vi "Refresh To Find New VIs.vi"(8 "error in":errorcluster, 10 "VIs  to exclude":variant, 11 "state in":T1) -> (0 "error out":errorcluster, 3 "state out":T1)   [LabVIEW 2010, in "NI_SE_Config Front Panel Layout.lvlib"]
uses:
  NI_SE_Config Front Panel Layout.lvlib
  State.ctl
  VI Info.ctl
  VI Panel Layout/VI Panel Layout.lvclass
  NI_SE_Front Panel Layout.lvlib
panel:
  in  "dummy object":dbl
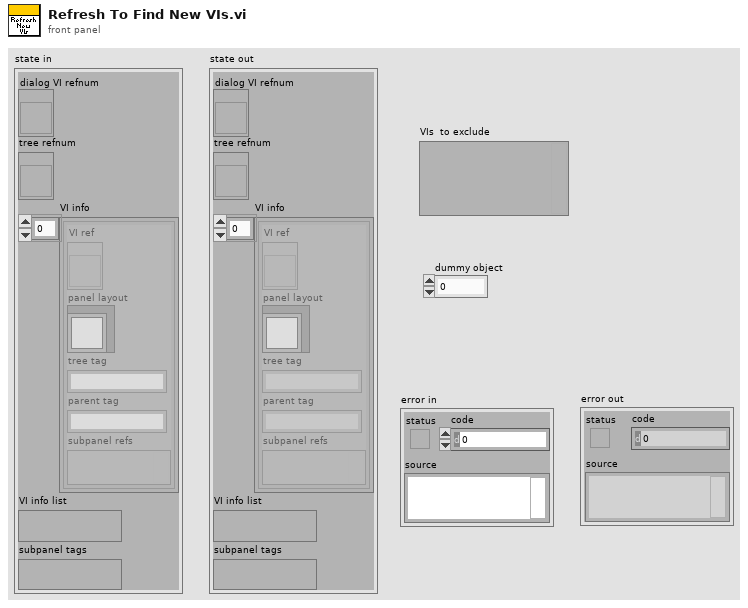
[diagram p1: front panel]
types:
  T1 = typedef "NI_SE_Config Front Panel Layout.lvlib/State.ctl" = cluster{"dialog VI refnum":refnum<vi>, "tree refnum":refnum<vi>, "VI info":T2[], "VI info list":variant, "subpanel tags":variant}
  T2 = typedef "NI_SE_Config Front Panel Layout.lvlib/VI Info.ctl" = cluster{"VI ref":refnum<vi>, "panel layout":refnum<class "VI Panel Layout.lvclass">, "tree tag":string, "parent tag":string, "subpanel refs":variant}
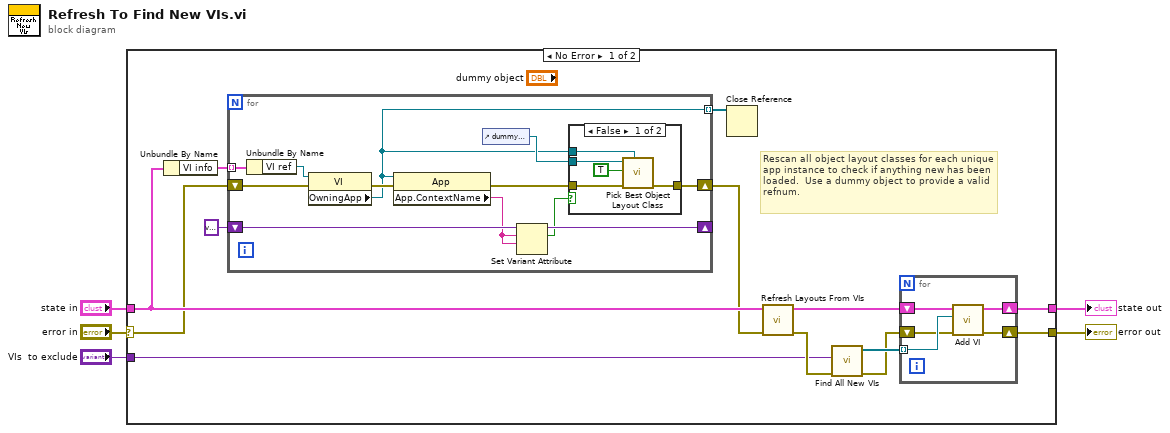
[diagram p0: block diagram]
diagram:
  n1 = case shown="No Error" "error in" {
    selector: "error in" -> [w8 w42]
    tunnel: "state in" -> [w11 w43]
    tunnel: [w13 w43] -> w3
    tunnel: [w12 w42] -> w2
    tunnel: "VIs  to exclude" -> [w14 _]
    frame No Error {
      # "Rescan all object layout classes for each unique app instance to check if anything new has been loaded.  Use a dummy object to provide a valid refnum."
      n2 = Unbundle By Name(w11) -> ("VI info"=w10:T2[])
      n3 = for {
        tunnel: w10 -> [w30] mode=indexing
        shift-right: [w28] -> _
        shift-left: variant -> [w27]
        shift-right: [w23] -> w7
        shift-left: w8 -> [w26]
        tunnel: [w19] -> w6 mode=indexing
        n4 = Unbundle By Name(w30) -> ("VI ref"=w29:refnum<vi>)
        n5 = property class="VI"(reference=w29, error in=w26) -> (error out=w22:errorcluster, "OwningApp"=w19:refnum<vi>)  [unwired: 1 out]
        n6 = property class="App"(reference=w19, error in=w22) -> (error out=w21:errorcluster, "App.ContextName"=w20:string)  [unwired: 1 out]
        n7 = control-ref of="dummy object"() -> (w24:refnum<vi>)
        n8 = Set Variant Attribute(Variant=w27, name=w20, value=w20) -> (Variant out=w28:variant, replaced=w25:bool)  [unwired: 1 in, 1 out]
        n9 = case shown="False" w25 {
          tunnel: w24 -> [w34 _]
          tunnel: w19 -> [w33 _]
          tunnel: w21 -> [w32 w36]
          tunnel: [w31 w36] -> w23
          frame False {
            n10 = call "Pick Best Object Layout Class.vi"("application reference"=w33, "error in"=w32, "rescan classes (F)"=TRUE ("rescan (F)"), "GObj Refnum"=w34) -> ("error out"=w31:errorcluster)  [unwired: 5 in, 2 out]
          }
          frame True {
          }
        }
      }
      n11 = Close Reference(reference=w6) -> ()  [unwired: 1 in, 1 out]
      n12 = call "Refresh Layouts From VIs.vi"("error in"=w7, "state in"=w11) -> ("error out"=w18:errorcluster, "state out"=w17:T1)  [unwired: 8 in]
      n13 = call "Find All New VIs.vi"("error in"=w18, "VIs  to exclude"=w14) -> ("error out"=w15:errorcluster, "VI refs"=w16:refnum<vi>[])  [unwired: 8 in]
      n14 = for {
        shift-right: [w40] -> w13
        shift-left: w17 -> [w41]
        tunnel: w16 -> [w39] mode=indexing
        shift-right: [w37] -> w12
        shift-left: w15 -> [w38]
        n15 = call "Add VI.vi"("error in"=w38, "VI ref"=w39, "state in"=w41) -> ("error out"=w37:errorcluster, "state out"=w40:T1)  [unwired: 7 in]
      }
    }
    frame Error {
    }
  }
  "state out" <- w3
  "error out" <- w2
